vi "Read 1s Buffer.vi"(8 "error in":errorcluster, 11 "CPC in":refnum<class "CPC.lvclass">) -> (0 "error out":errorcluster, 2 "1s Buff":i32, 3 "CPC out":refnum<class "CPC.lvclass">)   [LabVIEW 2014, in "CPC.lvclass"]
uses:
  CPC.lvclass
  CPC.lvclass/CPC.ctl
  reusable/Session APIs/Serial/Public/Get Data/Get Long Integer.vi
  reusable/Session APIs/Serial/Serial Session.lvclass
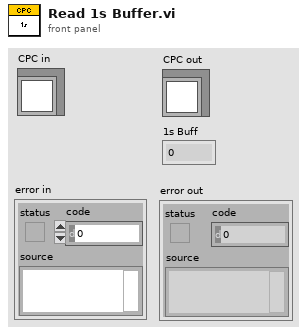
[diagram p1: front panel]
types:
  T1 = typedef "Serial Session.lvclass/Session Handle.ctl" = refnum<data-value>
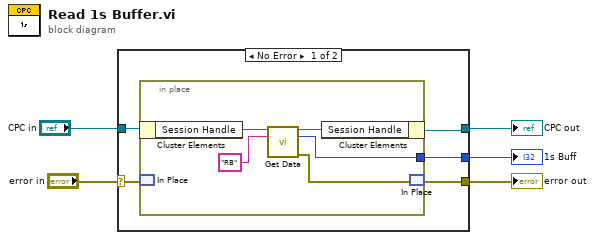
[diagram p0: block diagram]
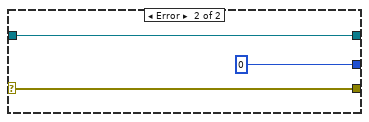
[diagram p2: hidden frame]
diagram:
  n1 = case shown="No Error" "error in" {
    selector: "error in" -> [w9 w18]
    tunnel: "CPC in" -> [w10 w17]
    tunnel: [w7 w18] -> w3
    tunnel: [w8 w17] -> w2
    tunnel: [w6 0 ("DataOut")] -> w4
    frame No Error {
      n2 = in-place {
        in-place-border: [w11] -> w6
        n3 = in-place-cluster #1(w10) -> ("Session Handle"=w15:T1)
        n4 = in-place-match #2(w9) -> ()  [unwired: 1 out]
        n5 = call-poly "Get Data.vi"("Session Handle in"=w15, "CMD"="RB" ("string")) -> ("Session Handle out"=w14:T1, "DataOut"=w11:i32, "error out"=w12:errorcluster)  [unwired: 11 in]
        n6 = in-place-cluster #1("Session Handle"=w14) -> (w8:refnum<class "CPC.lvclass">)
        n7 = in-place-match #2(w12) -> (w7:errorcluster)
      }
    }
    frame Error {
    }
  }
  "error out" <- w3
  "CPC out" <- w2
  "1s Buff" <- w4
